vi "Pretty Print.vi"(0 "JSON String":string) -> (1 "Invalid JSON":bool, 2 "Pretty JSON String":string)   [LabVIEW 2011, in "LV JSON.lvlib"]
doc: "Format JSON string with white space to make it readable.\n\nInvalid JSON boolean indicates when the input JSON string is missing a close bracket or close brace. (It does NOT check for valid JSON formatting.)"
uses:
  LV JSON.lvlib
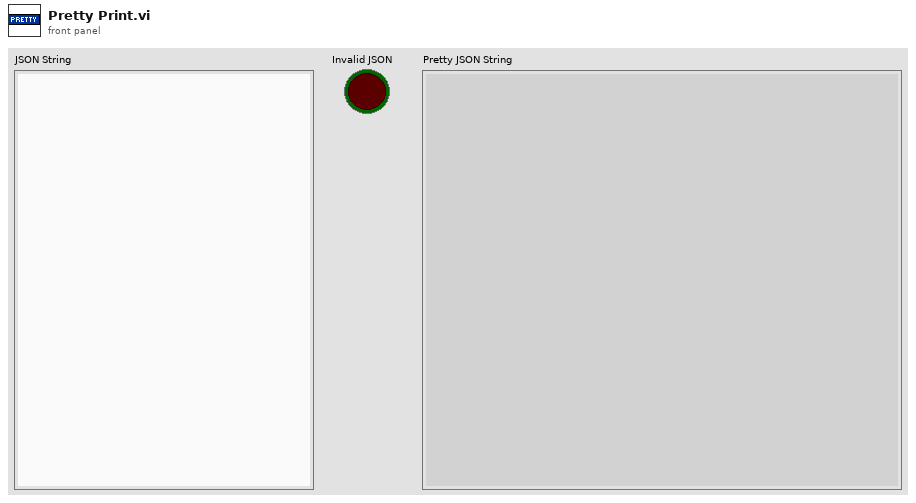
[diagram p1: front panel]
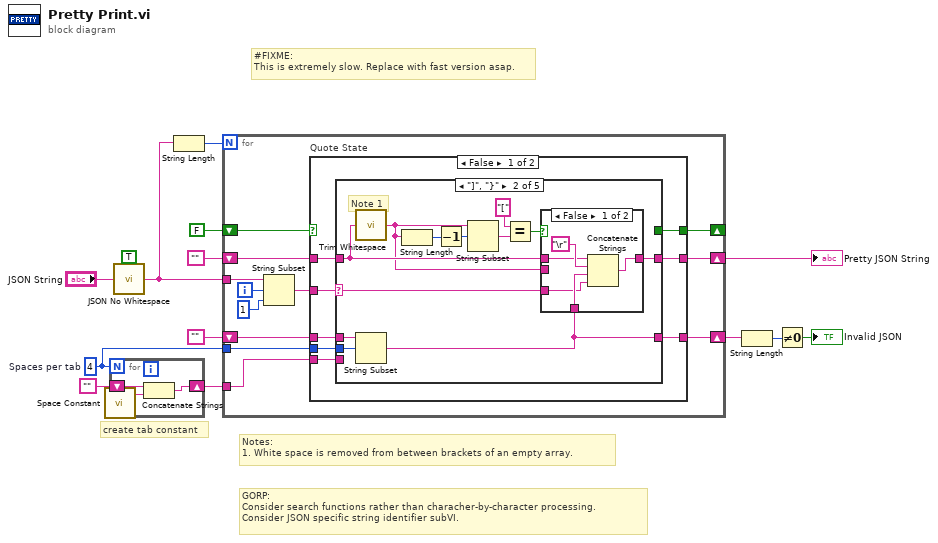
[diagram p0: block diagram]
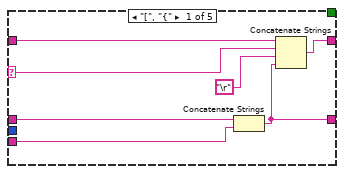
[diagram p2: hidden frame]
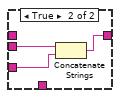
[diagram p3: hidden frame]
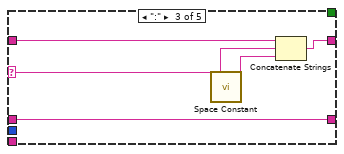
[diagram p4: hidden frame]
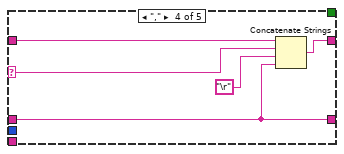
[diagram p5: hidden frame]
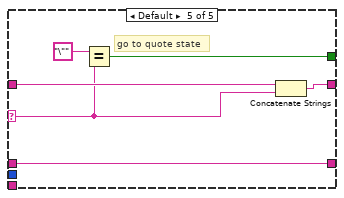
[diagram p6: hidden frame]
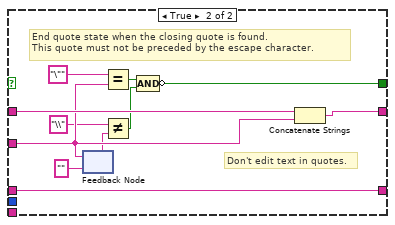
[diagram p7: hidden frame]
diagram:
  w10 = 4  # Spaces per tab
  # "#FIXME:\nThis is extremely slow. Replace with fast version asap."
  # "GORP:\nConsider search functions rather than characher-by-character processing.\nConsider JSON specific string identifier subVI."
  # "Notes:\n1. White space is removed from between brackets of an empty array."
  # "create tab constant"
  n1 = for {
    N: w10 -> [_]
    shift-right: [w16] -> w11
    shift-left: "" -> [w15]
    n2 = call <vilib>:"Space Constant.vi"() -> ("String"=w17:string)
    n3 = Concatenate Strings(w15, w17) -> (w16:string)
  }
  n4 = call "JSON No Whitespace.vi"("String"="JSON String", "Except in Quotes (F)"=TRUE) -> ("Trimmed String"=w3:string)
  n5 = String Length(string=w3) -> (length=w13:i32)
  n6 = for {
    N: w13 -> [_]
    shift-right: [w24] -> w7
    shift-left: "" ("Indent") -> [w26]
    tunnel: w3 -> [w27]
    tunnel: w11 -> [w25]
    tunnel: w10 -> [w23]
    shift-right: [w20] -> w8
    shift-left: "" -> [w21]
    shift-right: [w19] -> _
    shift-left: FALSE -> [w18]
    i -> [w29]
    n7 = String Subset(string=w27, offset (0)=w29, length (rest)=1 ("length (rest)")) -> (substring=w22:string)
    n8 = case "Quote State" shown="False" w18 {
      tunnel: w26 -> [w37 w88]
      tunnel: w25 -> [w36 _]
      tunnel: [w35 w88] -> w24
      tunnel: w23 -> [w34 _]
      tunnel: w22 -> [w33 w85]
      tunnel: w21 -> [w32 w90]
      tunnel: [w31 w89] -> w20
      tunnel: [w30 w87] -> w19
      frame False {
        n9 = case shown="\"]\", \"}\"" w33 {
          selector: w33 -> [w41 w52 w66 w72 w77]
          tunnel: [w40 w53 w69 w70 w80] -> w35
          tunnel: w37 -> [w44 w56 w69 w70 w80]
          tunnel: w36 -> [w43 _ _ _ _]
          tunnel: w34 -> [_ w55 _ _ _]
          tunnel: w32 -> [w42 w48 w67 w73 w79]
          tunnel: [w38 w54 w68 w74 w78] -> w31
          tunnel: [_ _ _ _ w75] -> w30
          frame "[", "{" {
            n10 = Concatenate Strings(w44, w43) -> (w40:string)
            n11 = Concatenate Strings(w42, w41, "\r", w40) -> (w38:string)
          }
          frame "]", "}" {
            # "Note 1"
            n12 = call <vilib>:"Trim Whitespace.vi"("string"=w48) -> ("trimmed string"=w46:string)  [unwired: 1 in]
            n13 = String Subset(string=w56, offset (0)=w55) -> (substring=w53:string)  [unwired: 1 in]
            n14 = String Length(string=w46) -> (length=w49:i32)
            n15 = Decrement(x=w49) -> (x-1=w45:i32)
            n16 = String Subset(string=w46, offset (0)=w45) -> (substring=w50:string)  [unwired: 1 in]
            n17 = Equal?(x="[", y=w50) -> (x = y?=w47:bool)
            n18 = case shown="False" w47 {
              tunnel: [w61 w64] -> w54
              tunnel: w53 -> [w60 _]
              tunnel: w52 -> [w59 w63]
              tunnel: w48 -> [w57 _]
              tunnel: w46 -> [_ w62]
              frame False {
                n19 = Concatenate Strings(w57, "\r", w60, w59) -> (w61:string)
              }
              frame True {
                n20 = Concatenate Strings(w62, w63) -> (w64:string)
              }
            }
          }
          frame ":" {
            n21 = call <vilib>:"Space Constant.vi"() -> ("String"=w65:string)
            n22 = Concatenate Strings(w67, w66, w65) -> (w68:string)
          }
          frame "," {
            n23 = Concatenate Strings(w73, w72, "\r", w70) -> (w74:string)
          }
          frame Default {
            # "go to quote state"
            n24 = Equal?(x="\"", y=w77) -> (x = y?=w75:bool)
            n25 = Concatenate Strings(w79, w77) -> (w78:string)
          }
        }
      }
      frame True {
        # "End quote state when the closing quote is found.\nThis quote must not be preceded by the escape character."
        # "Don't edit text in quotes."
        n26 = feedback-in #1(w85) -> ()
        n27 = feedback #1("" ("Trimmed String")) -> (w84:string)
        n28 = Equal?(x="\"", y=w85) -> (x = y?=w86:bool)
        n29 = Not Equal?(x="\\" ("Trimmed String"), y=w84) -> (x != y?=w82:bool)
        n30 = Compound Arithmetic op=AND(w86, w82) -> (invert w87:bool)
        n31 = Concatenate Strings(w90, w85) -> (w89:string)
      }
    }
  }
  "Pretty JSON String" <- w8
  n32 = String Length(string=w7) -> (length=w6:i32)
  n33 = Not Equal To 0?(x=w6) -> (x != 0?=→"Invalid JSON":bool)
